vi "Build Preview.vi"(7 "Ambient":dbl, 8 "error in (no error)":errorcluster, 9 "Start Temp":dbl, 10 "Start Time":dbl, 11 "Target Step in":refnum<class "Target Step.lvclass">) -> (0 "error out":errorcluster, 1 "End Temp":dbl, 2 "End Time":dbl, 3 "Target Step out":refnum<class "Target Step.lvclass">, 4 "Step Plot Data":cluster{"Time":dbl[], "Value":dbl[]})   [LabVIEW 2018, in "Temp Recipe.lvlib" / "Target Step.lvclass"]
uses:
  Target Step.lvclass
  Target Step.lvclass/Target Step.ctl
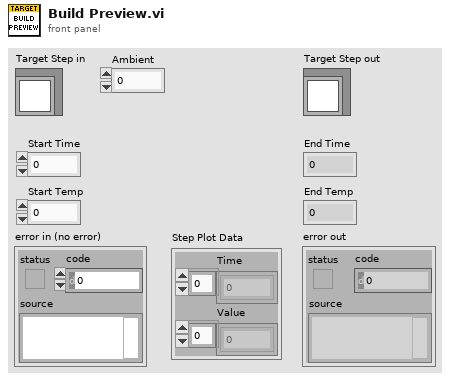
[diagram p1: front panel]
types:
  T1 = typedef "Temp Recipe.lvlib/Target Step.lvclass/Ref Data.ctl" = cluster{"Step Temp":dbl, "Settle Time":dbl}
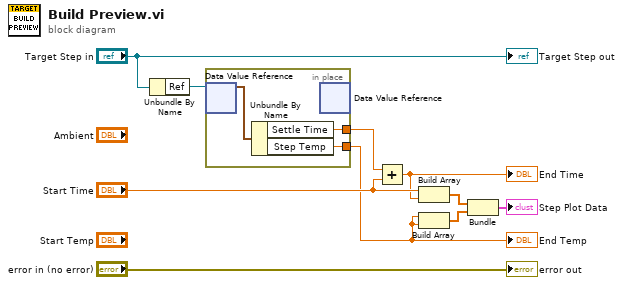
[diagram p0: block diagram]
diagram:
  n1 = Unbundle By Name("Target Step in") -> ("Ref"=w9:refnum<data-value>)
  n2 = in-place {
    in-place-border: [w12] -> w4
    in-place-border: [w11] -> w7
    n3 = in-place-dvr #1(w9) -> (w13:T1)  [unwired: 1 out]
    n4 = Unbundle By Name(w13) -> ("Settle Time"=w11:dbl, "Step Temp"=w12:dbl)
    n5 = in-place-dvr #1() -> ()  [unwired: 1 in, 2 out]
  }
  "End Temp" <- w4
  n6 = Add(x=w7, y="Start Time") -> (x+y=w5:dbl)
  "End Time" <- w5
  n7 = Build Array("Start Time", w5) -> (w3:dbl[])
  n8 = Build Array(w4, w4) -> (w2:dbl[])
  n9 = Bundle(w3, w2) -> (→"Step Plot Data":cluster{dbl[], dbl[]})  [unwired: 1 in]
  "error out" <- "error in (no error)"
  "Target Step out" <- "Target Step in"
